vi "EnqueueMessage(Single).vi"(6 "Priority Message? (F)":bool, 8 "error in (no error)":errorcluster, 9 "Message Data":variant, 10 "Message":string, 11 "Message Queue":refnum<queue>) -> (0 "error out":errorcluster, 3 "dup Message Queue":refnum<queue>)   [LabVIEW 2017, in "Server.lvlib" / "Message Queue.lvlib"]
doc: "For a regular message, enqueue the message. For a priority message, enqueue it at the front of the queue."
uses:
  Message Queue.lvlib
  MessageCluster.ctl
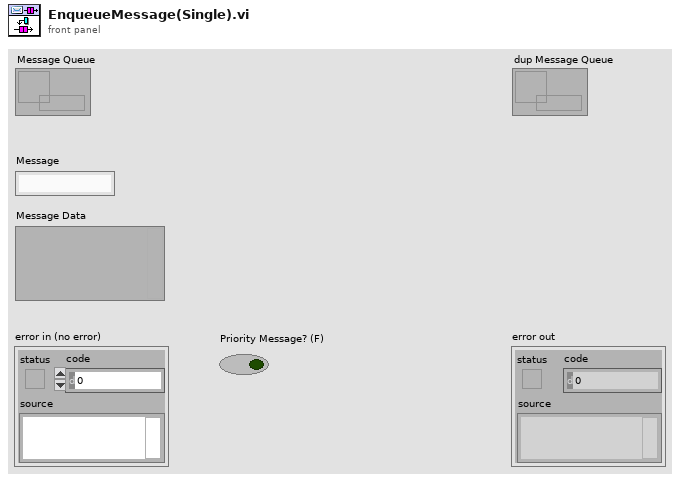
[diagram p1: front panel]
types:
  T1 = typedef "Server.lvlib/Message Queue.lvlib/MessageCluster.ctl" = cluster{"Message":string, "Message Data":variant}
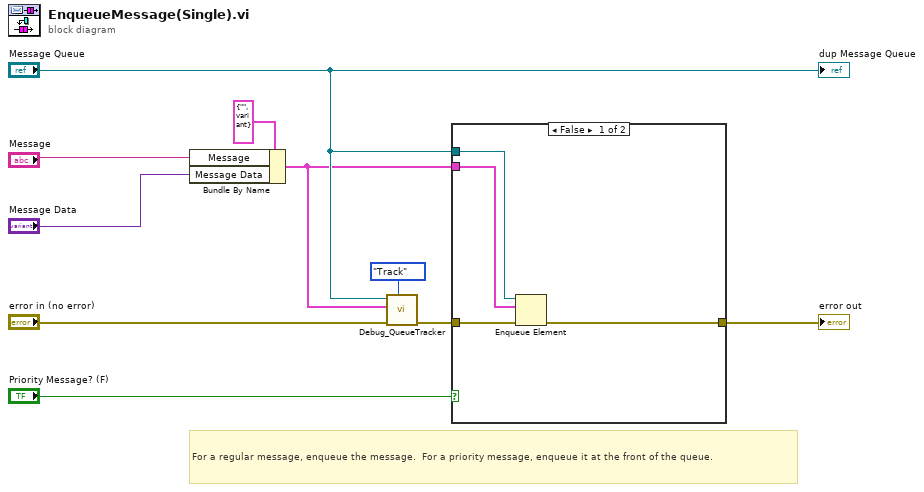
[diagram p0: block diagram]
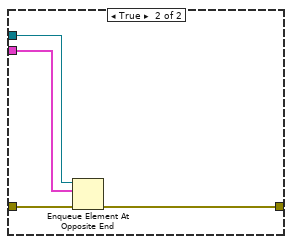
[diagram p2: hidden frame]
diagram:
  # "For a regular message, enqueue the message.  For a priority message, enqueue it at the front of the queue."
  n1 = Bundle By Name(cluster=T1 {"Message"="", "Message Data"=variant} ("Message Cluster"), "Message"="Message", "Message Data"="Message Data") -> (w2:T1)
  n2 = call "Debug_QueueTracker.vi"("Mode"=enum16{"Init", "Track", "DeInit"}."Track", "Error In"="error in (no error)", "Message Cluster"=w2, "QueueIn"="Message Queue") -> ("Error Out"=w4:errorcluster)  [unwired: 7 in]
  n3 = case shown="False" "Priority Message? (F)" {
    tunnel: w4 -> [w14 w18]
    tunnel: [w13 w17] -> w5
    tunnel: "Message Queue" -> [w12 w16]
    tunnel: w2 -> [w11 w15]
    frame False {
      n4 = Enqueue Element(queue=w12, element=w11, error in (no error)=w14) -> (error out=w13:errorcluster)  [unwired: 1 in, 2 out]
    }
    frame True {
      n5 = Enqueue Element At Opposite End(queue=w16, element=w15, error in (no error)=w18) -> (error out=w17:errorcluster)  [unwired: 1 in, 2 out]
    }
  }
  "error out" <- w5
  "dup Message Queue" <- "Message Queue"
